vi "set Player Type.vi"(10 "Player Type":T1, 11 "Element in":refnum<class "Element.lvclass">) -> (3 "Element out":refnum<class "Element.lvclass">)   [LabVIEW 2021, in "Element.lvclass"]
uses:
  Element.lvclass
  Element.lvclass/Element.ctl
  Player Type.ctl
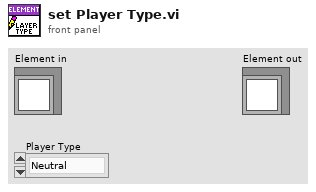
[diagram p1: front panel]
types:
  T1 = typedef "Element.lvclass/Player Type.ctl" = enum16{"Neutral", "Player 1", "Player 2"}
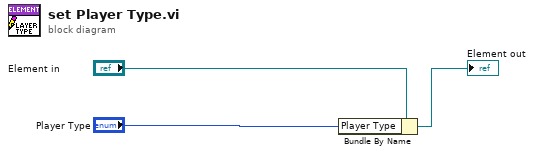
[diagram p0: block diagram]
diagram:
  n1 = Bundle By Name(cluster="Element in", "Player Type"="Player Type") -> (→"Element out":refnum<class "Element.lvclass">)
